vi "Pack for gRPC.vi"(8 "error in":errorcluster, 9 "configuration / results":enum16{"Configuration", "Results"}(ring), 10 "data value":variant, 11 "measurement customizations in":refnum<class "Measurement Plugin.lvclass">) -> (0 "error out":errorcluster, 2 "any":T1, 3 "measurement customizations out":refnum<class "Measurement Plugin.lvclass">)   [LabVIEW 2022 SP3, in "Single Tone - Digital Mic.lvlib" / "Measurement Plugin.lvclass"]
uses:
  Measurement Plugin.lvclass
  <vilib>/gRPC/LabVIEW gRPC Library/Shared/Any.ctl
  C:/Program Files/National Instruments/LabVIEW 2022/vi.lib/Plug-In SDKs/Measurements/Measurement Plugin Service/Measurement Plugin Service.lvclass
  Measurement Configuration.ctl
  shared/measurements/controls/lowpass filter.ctl
  shared/measurements/controls/weighting filter.ctl
  shared/measurements/controls/highpass filter.ctl
  shared/measurements/controls/measurement units.ctl
  Measurement Results.ctl
  2eca732d-dbaa-43bf-a7dd-ede2da65bc1b.vi
  a6012965-5700-4384-8228-972e71b6560c.vi
  <vilib>/gRPC/LabVIEW gRPC Library/Server API/Translate Protobuf Error.vi
  <vilib>/AdvancedString/1D String Array to Delimited String.vi
  <vilib>/gRPC/LabVIEW gRPC Library/Server API/Server/Get Server DLL Path.vi
  Single Tone - Digital Mic.lvlib
  <vilib>/Plug-In SDKs/Measurements/Measurement Plugin Service/Measurement Plugin Service.lvclass
  <vilib>/gRPC/LabVIEW gRPC Library/grpc-lvsupport-release.lvlib
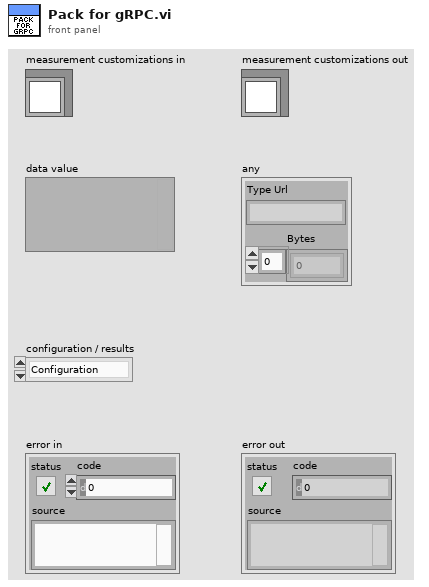
[diagram p1: front panel]
types:
  T1 = typedef "grpc-lvsupport-release.lvlib/Any.ctl" = cluster{"Type Url":string, "Bytes":u8[]}
  T2 = typedef "grpc-lvsupport-release.lvlib/grpcId.ctl" = u64
  T3 = typedef "Single Tone - Digital Mic.lvlib/Measurement Configuration.ctl" = cluster{"digital channel list":string, "input cfg file":string, "digital mic sensitivity (dBFS)":dbl, "ref mic channel":string, "ref mic sensitivity (mV/Pa)":dbl, "output channel":string, "signal frequency":dbl, "output level (dBSPL)":dbl, "output voltage ratio":dbl, "lowpass filter":T4, "weighting filter":T5, "highpass filter":T6, "band start":dbl, "band stop":dbl, "min measurement cycles":u32, "min measurement time (s)":dbl, "min settling cycles":u32, "min settling time (s)":dbl, "SNR units":T7, "THD+N units":T7, "THD units":T7}
  T4 = typedef "lowpass filter.ctl" = enum32{"No filter", "AES17 20kHz", "AES17 40kHz"}
  T5 = typedef "weighting filter.ctl" = enum32{"Linear", "A-weighting", "B-weighting", "C-weighting"}
  T6 = typedef "highpass filter.ctl" = enum32{"DC", "AC"}
  T7 = typedef "measurement units.ctl" = enum32{"dB", "%", "x/y"}
  T8 = typedef "Single Tone - Digital Mic.lvlib/Measurement Results.ctl" = cluster{"channel name":string, "frequency (Hz)":dbl, "amplitude (Pa RMS)":dbl, "amplitude (dBSPL)":dbl, "microphone sensitivity (dBFS)":dbl, "SNR":dbl, "THD+N":dbl, "THD":dbl, "wfm - dt":dbl, "wfm - data":dbl[], "fft - f0":dbl, "fft - df":dbl, "fft - data":dbl[], "ref mic wfm - dt":dbl, "ref mic wfm - data":dbl[]}
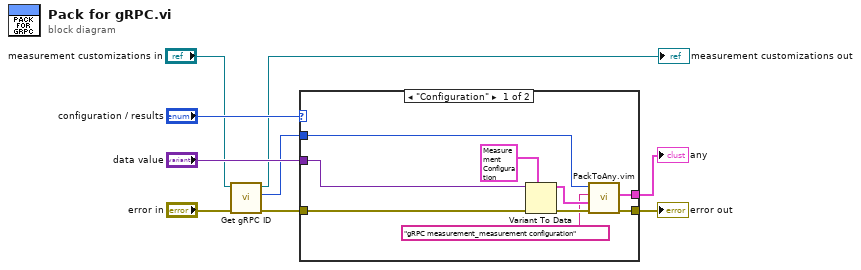
[diagram p0: block diagram]
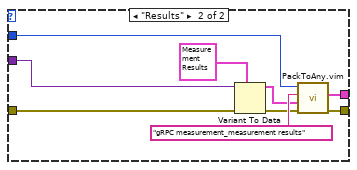
[diagram p2: hidden frame]
diagram:
  n1 = call <vilib>:"Get gRPC ID.vi"("error in"="error in", "measurement plugin service in"="measurement customizations in") -> ("error out"=w4:errorcluster, "gRPC ID"=w1:T2, "measurement plugin service out"=→"measurement customizations out":refnum<class "Measurement Plugin.lvclass">)  [unwired: 7 in]
  n2 = case shown="\"Configuration\"" "configuration / results" {
    tunnel: w4 -> [w18 w27]
    tunnel: "data value" -> [w17 w26]
    tunnel: w1 -> [w14 w22]
    tunnel: [w16 w24] -> w8
    tunnel: [w15 w23] -> w7
    frame "Configuration" {
      n3 = Variant To Data(error in=w18, type=T3 {"digital channel list"="Lorem ipsum dolor sit", "input cfg file"="", "digital mic sensitivity (dBFS)"=1.2, "ref mic channel"="7821\\PCMo 0", "ref mic sensitivity (mV/Pa)"=32.0, "output channel"="7821\\PCMo 0", "signal frequency"=64.0, "output level (dBSPL)"=-32.0, "output voltage ratio"=-64.0, "lowpass filter"=enum."No filter", "weighting filter"=enum."A-weighting", "highpass filter"=enum."AC", "band start"=1.0, "band stop"=1.0, "min measurement cycles"=20, "min measurement time (s)"=0.1, "min settling cycles"=0, "min settling time (s)"=0.0, "SNR units"=enum."dB", "THD+N units"=enum."dB", "THD units"=enum."dB"} ("measurement configuration"), Variant=w17) -> (data=w13:T3, error out=w12:errorcluster)
      n4 = call "PackToAny.vim"("error in"=w12, "Data To Pack"=w13, "Message Type"="gRPC measurement_measurement configuration", "gRPCid in"=w14) -> ("error out"=w16:errorcluster, "Any"=w15:T1)  [unwired: 5 in, 1 out]
    }
    frame "Results" {
      n5 = Variant To Data(error in=w27, type=T8 {"channel name"="Empty", "frequency (Hz)"=0.0, "amplitude (Pa RMS)"=0.0, "amplitude (dBSPL)"=0.0, "microphone sensitivity (dBFS)"=0.0, "SNR"=0.0, "THD+N"=0.0, "THD"=0.0, "wfm - dt"=0.0, "wfm - data"=[], "fft - f0"=0.0, "fft - df"=0.0, "fft - data"=[], "ref mic wfm - dt"=0.0, "ref mic wfm - data"=[]} ("Measurement Results"), Variant=w26) -> (data=w20:T8, error out=w19:errorcluster)
      n6 = call "PackToAny.vim"("error in"=w19, "Data To Pack"=w20, "Message Type"="gRPC measurement_measurement results", "gRPCid in"=w22) -> ("error out"=w24:errorcluster, "Any"=w23:T1)  [unwired: 5 in, 1 out]
    }
  }
  "error out" <- w8
  "any" <- w7
